vi "RunMeas.vi"(8 "error in (no error)":errorcluster, 11 "ChromaPowerSupplyModel in":refnum<class "ChromaPowerSupplyModel.lvclass">) -> (0 "error out":errorcluster, 2 "variant":variant, 3 "ChromaPowerSupplyModel out":refnum<class "ChromaPowerSupplyModel.lvclass">)   [LabVIEW 2018, in "AcPwrPlugins.lvlib" / "ChromaPowerSupplyModel.lvclass"]
doc: "This VI initiates and takes measurements from the instrument(s)."
uses:
  ChromaPowerSupplyModel.lvclass
  AcPwrShared/clMeasurmentData.ctl
  AcPwrShared/clAcPwrAttributes.ctl
  AcPwrShared/clEventType.ctl
  AcPwrShared/AcPwrShared.lvlib
  AcPwrBaseClass/AcPwrBase.lvclass
panel:
  out "Waveform Chart":waveform(dbl)[](graph)
  in  "Measure Type (Voltage)":i32(ring) items=["Voltage", "Current", "Power"]
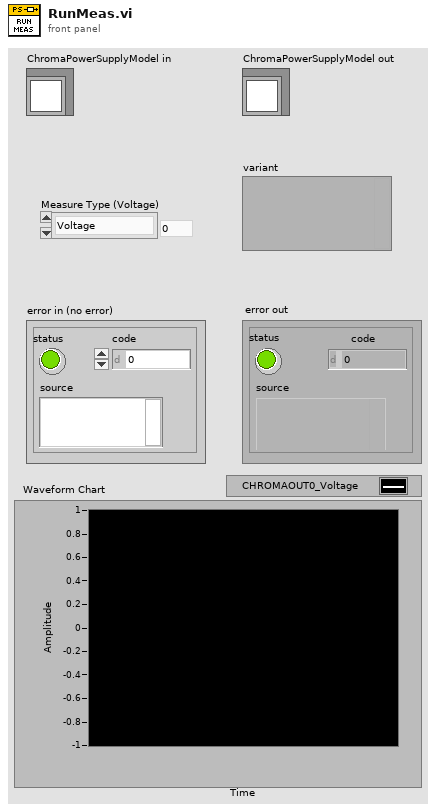
[diagram p1: front panel]
types:
  T1 = typedef "AcPwrPlugins.lvlib/ChromaPowerSupply.lvclass/Measurements.ctl" = cluster{"Handle":string, "Name":string, "Enabled":bool, "Measurement Value":dbl, "btnMeasFetch":bool, "ProtectionStatusString":string, "Measurement Type":enum16{"Voltage", "Current", "Power"}}[]
  T2 = typedef "AcPwrPlugins.lvlib/ChromaPowerSupply.lvclass/Device(s)Settings.ctl" = cluster{"Phases":cluster{"Handle":string, "Instrument Options":string, "id query (T)":bool, "reset device (T)":bool, "Timing":cluster{"TimingOn":enum16{""}, "Hours":u32, "Minutes":u32, "Seconds":dbl, "CutoffVoltage":dbl}, "Connected":bool, "Output Mode":enum16{"Voltage (DC)", "Current (DC)"}, "Voltage":dbl, "Current":dbl, "High Voltage Limit":dbl, "High Current Limit":dbl, "Power Protect":dbl, "Current Protect":dbl, "Voltage Protect":dbl, "Low Current Limit":dbl, "Low Voltage Limit":dbl, "Current Slew Rate":dbl, "Voltage Slew Rate":dbl}[], "MeasName":string}
  T3 = typedef "AcPwrShared.lvlib/clMeasurmentData.ctl" = cluster{"MeasName":string, "XML Data":string, "WaveformData":waveform(dbl)[]}
  T4 = typedef "AcPwrShared.lvlib/clEventType.ctl" = cluster{"ModuleID":i32, "Data":variant}
  T5 = typedef "AcPwrPlugins.lvlib/ChromaPowerSupplyModel.lvclass/ChromaPS_Model2ICDAS.ctl" = cluster{"data_id":i32, "voltage":dbl, "current":dbl, "power":dbl, "meas_timestamp":timestamp, "write_timestamp":timestamp, "read_by_icdas":bool, "read_timestamp":timestamp}
  T6 = typedef "AcPwrShared.lvlib/clAcPwrAttributes.ctl" = cluster{"ProtectionStatusString":string, "Handle_MeasurementType":string, "Status Byte Register":cluster{"Busy":bool, "Remote Mode":bool, "Error in Queue":bool, "QUES=Questionable Status Summary":bool, "MAV = Message Available":bool, "ESB = Event Status Byte Summary":bool, "RQS = Request for Service":bool, "OPER = Operation Event Summary":bool}}
  T7 = cluster{"Handle":string, "Name":string, "Enabled":bool, "Measurement Value":dbl, "btnMeasFetch":bool, "ProtectionStatusString":string, "Measurement Type":enum16{"Voltage", "Current", "Power"}}
  T8 = typedef "AcPwrShared.lvlib/AcPwrBroadcastEvents.ctl" = cluster{"DidInit":refnum<user-event>, "StatusUpdate":refnum<user-event>, "ErrorReport":refnum<user-event>, "DidStop":refnum<user-event>, "PathToINI":refnum<user-event>, "Measurements":refnum<user-event>, "LoadConfigFile":refnum<user-event>, "GetSettings":refnum<user-event>, "SetSettings":refnum<user-event>, "GetType&ID":refnum<user-event>, "GotSettings":refnum<user-event>, "GotSettingsLV":refnum<user-event>}
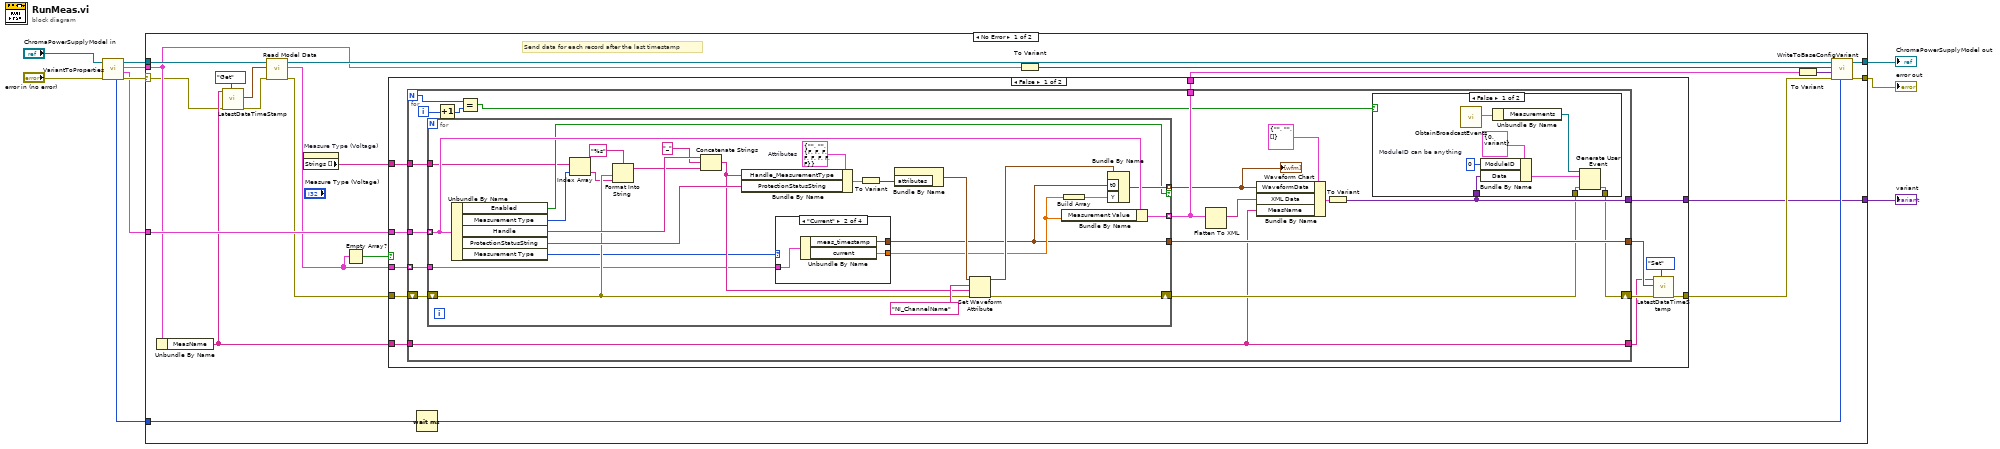
[diagram p0: block diagram]
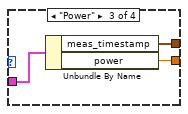
[diagram p4: hidden frame]
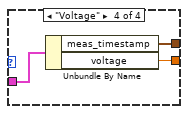
[diagram p5: hidden frame]
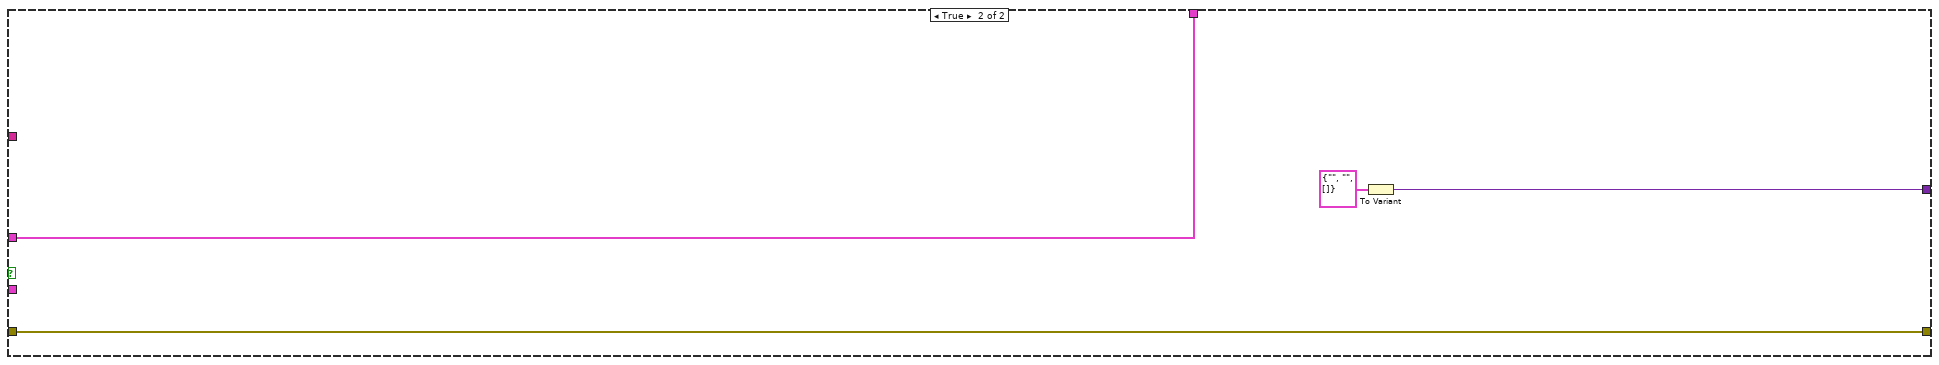
[diagram p6: hidden frame]
diagram:
  n1 = call "VariantToProperties.vi"("error in (no error)"="error in (no error)", "ChromaPowerSupplyModel in"="ChromaPowerSupplyModel in") -> ("error out"=w9:errorcluster, "Measurements"=w8:T1, "Device Settings"=w7:T2, "ChromaPowerSupplyModel out"=w10:refnum<class "ChromaPowerSupplyModel.lvclass">, "Measurement Refresh Time (ms)"=w6:u32)  [unwired: 4 in, 1 out]
  n2 = case shown="No Error" w9 {
    selector: w9 -> [w13 w111]
    tunnel: [w30 w112] -> w3
    tunnel: [w28 w111] -> w2
    tunnel: w10 -> [w20 w112]
    tunnel: w7 -> [w18 _]
    tunnel: w8 -> [w32 _]
    tunnel: w6 -> [w26 _]
    tunnel: [w23 _] -> w4
    frame No Error {
      # "Send data for each record after the last timestamp"
      n3 = Unbundle By Name(w18) -> ("MeasName"=w14:string)
      n4 = call "LatestDataTimeStamp.vi"("Action"=enum16{"Set", "Get"}."Get", "error in (no error)"=w13, "Plugin Name"=w14) -> ("error IO"=w12:errorcluster, "Latest Data Timestamp"=w11:timestamp)  [unwired: 6 in, 1 out]
      n5 = call "Read Model Data.vi"("error in (no error)"=w12, "meas_timestamp in"=w11, "ChromaPowerSupplyModel in"=w20) -> ("error out"=w19:errorcluster, "ICDAS2Model Data"=w17:T5[], "ChromaPowerSupplyModel out"=w21:refnum<class "ChromaPowerSupplyModel.lvclass">)  [unwired: 6 in]
      n6 = property on="Measure Type (Voltage)" class="Ring (strict)"() -> ("Strings []"=w22:string[])  [unwired: 2 in, 2 out]
      n7 = Empty Array?(array=w17) -> (empty?=w16:bool)
      n8 = case shown="False" w16 {
        tunnel: w32 -> [w44 w107]
        tunnel: [w36 w108] -> w31
        tunnel: [w43 w107] -> w24
        tunnel: w14 -> [w42 _]
        tunnel: [w41 w109] -> w23
        tunnel: w22 -> [w40 _]
        tunnel: w19 -> [w39 w108]
        tunnel: w17 -> [w38 _]
        frame False {
          n9 = for {
            N -> [w49]
            tunnel: w44 -> [w62]
            tunnel: [w61] -> w43
            tunnel: w42 -> [w45]
            tunnel: [w52] -> w41
            tunnel: w40 -> [w56]
            tunnel: [w54] -> w35
            shift-right: [w47] -> w37
            shift-left: w39 -> [w55]
            tunnel: w38 -> [w53] mode=indexing
            tunnel: [w45] -> w34
            i -> [w51]
            n10 = for {
              tunnel: w62 -> [w97] mode=indexing
              shift-right: [w76] -> w48
              shift-left: w55 -> [w80]
              tunnel: [w96] -> w61 mode=indexing
              tunnel: [w94] -> w57 mode=indexing if=w88
              tunnel: w56 -> [w79]
              tunnel: w53 -> [w74]
              tunnel: [w72] -> w54
              w87 = T6 {"ProtectionStatusString"="", "Handle_MeasurementType"="", "Status Byte Register"={"Busy"=FALSE, "Remote Mode"=FALSE, "Error in Queue"=FALSE, "QUES=Questionable Status Summary"=FALSE, "MAV = Message Available"=FALSE, "ESB = Event Status Byte Summary"=FALSE, "RQS = Request for Service"=FALSE, "OPER = Operation Event Summary"=FALSE}}  # Attributes
              n11 = Unbundle By Name(w97) -> ("Enabled"=w88:bool, "Measurement Type"=w77:enum16{"Voltage", "Current", "Power"}, "Handle"=w91:string, "ProtectionStatusString"=w85:string, "Measurement Type"=w75:enum16{"Voltage", "Current", "Power"})
              n12 = Index Array(array=w79, index=w77) -> (element=w78:string)
              n13 = Format Into String(format string="%s", error in=w80, w78) -> (resulting string=w89:string)  [unwired: 1 in, 1 out]
              n14 = Concatenate Strings(w91, "_", w89) -> (w82:string)
              n15 = Bundle By Name(cluster=w87, "Handle_MeasurementType"=w82, "ProtectionStatusString"=w85) -> (w86:T6)
              n16 = case shown="\"Current\"" w75 {
                tunnel: w74 -> [_ w100 w103 w106]
                tunnel: [_ w99 w102 w105] -> w72
                tunnel: [_ w98 w101 w104] -> w73
                frame Default {
                }
                frame "Current" {
                  n17 = Unbundle By Name(w100) -> ("meas_timestamp"=w99:timestamp, "current"=w98:dbl)
                }
                frame "Power" {
                  n18 = Unbundle By Name(w103) -> ("meas_timestamp"=w102:timestamp, "power"=w101:dbl)
                }
                frame "Voltage" {
                  n19 = Unbundle By Name(w106) -> ("meas_timestamp"=w105:timestamp, "voltage"=w104:dbl)
                }
              }
              n20 = To Variant(anything=w86) -> (Variant=w92:variant)
              n21 = Bundle By Name("attributes"=w92) -> (w81:waveform(dbl))  [unwired: 1 in]
              n22 = Set Waveform Attribute(4:w80, 5:w82, 6:"NI_ChannelName" ("name"), 7:w81) -> (0:w76:errorcluster, 3:w83:waveform(dbl))  [unwired: 1 out]
              n23 = Bundle By Name(cluster=w97, "Measurement Value"=w73) -> (w96:T7)
              n24 = Build Array(w73) -> (w95:dbl[])
              n25 = Bundle By Name(cluster=w83, "t0"=w72, "Y"=w95) -> (w94:waveform(dbl))
            }
            "Waveform Chart" <- w57
            n26 = Increment(x=w51) -> (x+1=w50:i32)
            n27 = Equal?(x=w49, y=w50) -> (x = y?=w46:bool)
            n28 = Flatten To XML(anything=w61) -> (xml string=w58:string)
            n29 = Bundle By Name(cluster=T3 {"MeasName"="", "XML Data"="", "WaveformData"=[]} ("MeasurmentDataCluster"), "WaveformData"=w57, "XML Data"=w58, "MeasName"=w45) -> (w59:T3)
            n30 = To Variant(anything=w59) -> (Variant=w52:variant)
            n31 = case shown="False" w46 {
              tunnel: w52 -> [w65 _]
              tunnel: w48 -> [w64 w71]
              tunnel: [w63 w71] -> w47
              frame False {
                w66 = 0  # ModuleID can be anything
                n32 = call "ObtainBroadcastEvents.vi"() -> ("AcPwrEvents"=w68:T8)  [unwired: 10 in, 1 out]
                n33 = Bundle By Name(cluster=T4 {"ModuleID"=0, "Data"=variant} ("clEventType"), "ModuleID"=w66, "Data"=w65) -> (w69:T4)
                n34 = Unbundle By Name(w68) -> ("Measurements"=w67:refnum<user-event>)
                n35 = Generate User Event(user event=w67, event data cluster=w69, error in=w64) -> (error out=w63:errorcluster)  [unwired: 1 in, 1 out]
              }
              frame True {
                # "Don't broadcast results for the last DB Record. The module should broadcast it after this VI is done."
              }
            }
          }
          n36 = call "LatestDataTimeStamp.vi"("Action"=enum16{"Set", "Get"}."Set", "error in (no error)"=w37, "TimeStamp"=w35, "Plugin Name"=w34) -> ("error IO"=w36:errorcluster)  [unwired: 5 in, 2 out]
        }
        frame True {
          n37 = To Variant(anything=T3 {"MeasName"="", "XML Data"="", "WaveformData"=[]} ("MeasurmentDataCluster")) -> (Variant=w109:variant)
        }
      }
      n38 = Wait (ms)(milliseconds to wait=w26) -> (millisecond timer value=w25:u32)
      n39 = To Variant(anything=w18) -> (Variant=w27:variant)
      n40 = To Variant(anything=w24) -> (Variant=w29:variant)
      n41 = call-dynamic "WriteToBaseConfigVariant.vi"("Measurement Refresh Time (ms)"=w25, "error in (no error)"=w31, "Meas"=w29, "Config"=w27, "ChromaPowerSupplyModel in"=w21) -> ("error out"=w28:errorcluster, "ChromaPowerSupplyModel out"=w30:refnum<class "ChromaPowerSupplyModel.lvclass">)  [unwired: 5 in]
    }
    frame Error {
    }
  }
  "ChromaPowerSupplyModel out" <- w3
  "error out" <- w2
  "variant" <- w4
